vi "sigmoid_v1.1.vi"(1 "x":T1) -> (0 "y":T1)   [LabVIEW 2020]
uses:
  <vilib>/Analysis/Matrix/Datatypes/RealMatrix.ctl
  <vilib>/Analysis/Matrix/Numeric/Conversions/Matrix To Array - RM.vi
  <vilib>/Analysis/Matrix/Numeric/Conversions/Array To Matrix - RA.vi
  <vilib>/Analysis/Matrix/NI_Matrix.lvlib
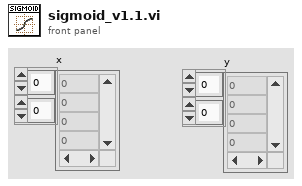
[diagram p1: front panel]
types:
  T1 = typedef "NI_Matrix.lvlib/RealMatrix.ctl" = dbl[][]
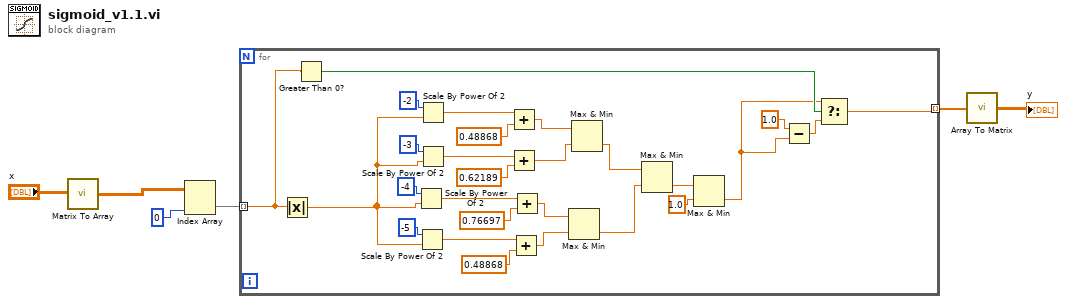
[diagram p0: block diagram]
diagram:
  n1 = call-poly <vilib>:"Matrix To Array.vi"("Real Matrix"="x") -> ("Real 2D Array"=w1:dbl[][])
  n2 = Index Array(array=w1, index (col)=0) -> (element=w4:dbl[])  [unwired: 1 in]
  n3 = for {
    tunnel: w4 -> [w12] mode=indexing
    tunnel: [w10] -> w3 mode=indexing
    n4 = Absolute Value(x=w12) -> (abs(x)=w29:dbl)
    n5 = Greater Than 0?(x=w12) -> (x > 0?=w11:bool)
    n6 = Scale By Power Of 2(n=-4, x=w29) -> (x*2^n=w23:dbl)
    n7 = Scale By Power Of 2(n=-5, x=w29) -> (x*2^n=w24:dbl)
    n8 = Scale By Power Of 2(n=-2, x=w29) -> (x*2^n=w21:dbl)
    n9 = Scale By Power Of 2(n=-3, x=w29) -> (x*2^n=w22:dbl)
    n10 = Add(x=w21, y=0.48868) -> (x+y=w20:dbl)
    n11 = Add(x=w22, y=0.62189) -> (x+y=w19:dbl)
    n12 = Add(x=w24, y=0.48868) -> (x+y=w17:dbl)
    n13 = Add(x=w23, y=0.76697) -> (x+y=w18:dbl)
    n14 = Max & Min(x=w18, y=w17) -> (min(x,y)=w15:dbl)  [unwired: 1 out]
    n15 = Max & Min(x=w20, y=w19) -> (min(x,y)=w16:dbl)  [unwired: 1 out]
    n16 = Max & Min(x=w16, y=w15) -> (min(x,y)=w9:dbl)  [unwired: 1 out]
    n17 = Max & Min(x=w9, y=1.0) -> (min(x,y)=w7:dbl)  [unwired: 1 out]
    n18 = Subtract(x=1.0, y=w7) -> (x-y=w13:dbl)
    n19 = Select(t=w7, s=w11, f=w13) -> (s? t:f=w10:dbl)
  }
  n20 = call-poly <vilib>:"Array To Matrix.vi"("Real 1D Array"=w3) -> ("Real Matrix (Column Vector)"=→"y":T1)
